vi "Get Hand Info p2.vi"(10 "Bid":u64, 11 "Hand":string) -> (3 "Hand Info":T1)   [LabVIEW 2023, in "d7.lvlib"]
uses:
  d7.lvlib
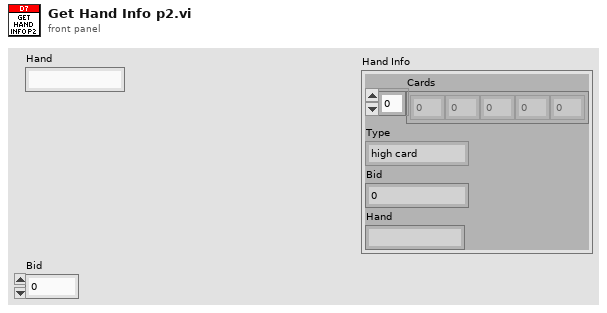
[diagram p1: front panel]
types:
  T1 = cluster{"Cards":i32[], "Type":enum16{"high card", "pair", "two pair", "3 of a kind", "full house", "4 of a kind", "5 of a kind"}, "Bid":u64, "Hand":string}
  T2 = enum16{"high card", "pair", "two pair", "3 of a kind", "full house", "4 of a kind", "5 of a kind"}
  T3 = cluster{i32[], enum16{"high card", "pair", "two pair", "3 of a kind", "full house", "4 of a kind", "5 of a kind"}, "Bid":u64, "Hand":string}
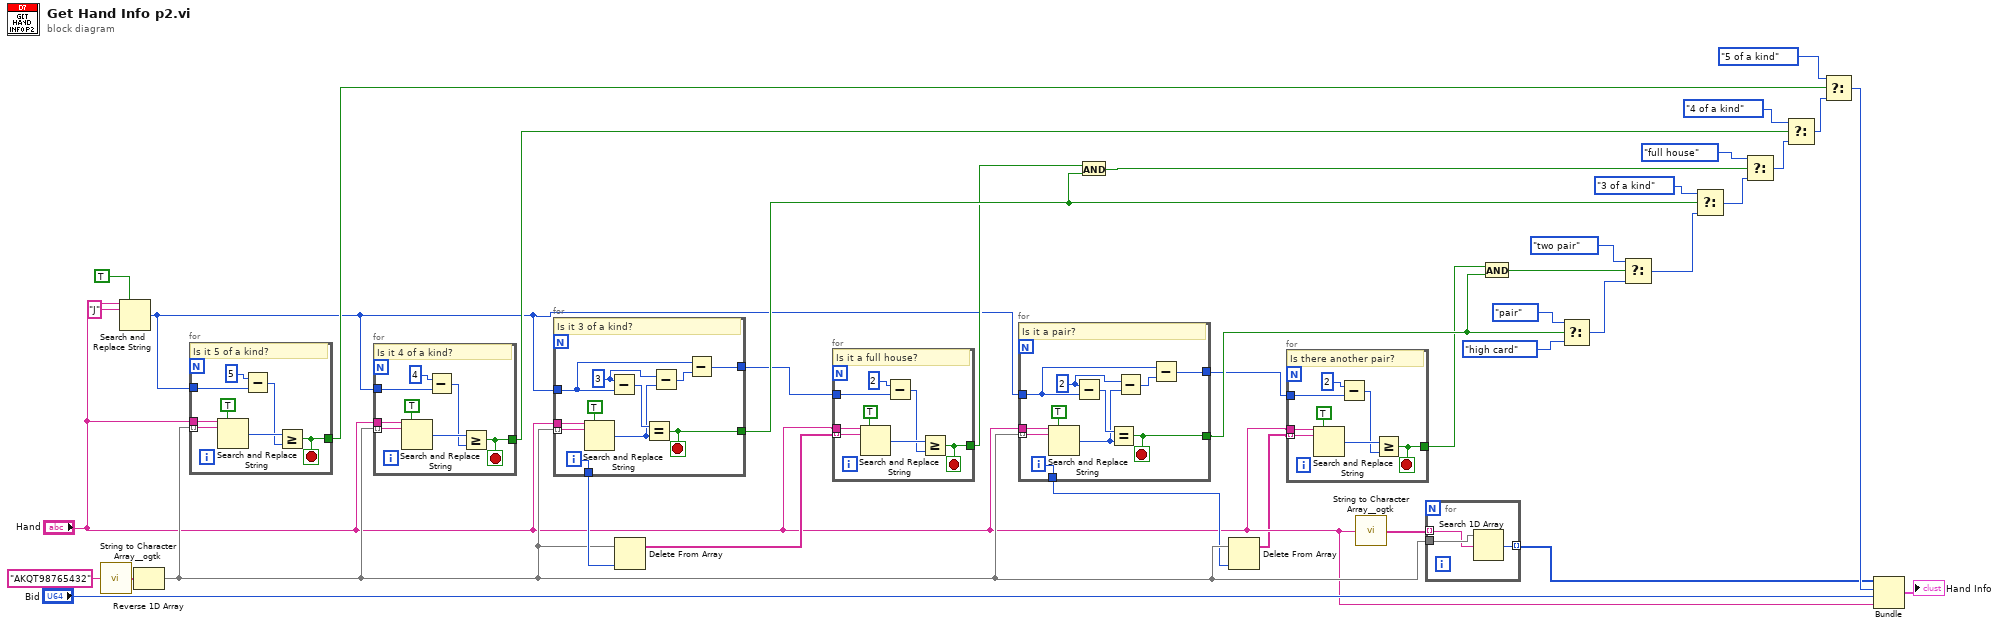
[diagram p0: block diagram]
diagram:
  n1 = call <userlib>:"String to Character Array__ogtk.vi"("Input String"="AKQT98765432" ("regular expression")) -> ("Character Array"=w27:string[])
  n2 = Search and Replace String(replace all?=TRUE ("replace all? (F)"), input string="Hand", search string="J" ("replace string (\"\")")) -> (number of replacements=w8:i32)  [unwired: 5 in, 3 out]
  n3 = Reverse 1D Array(array=w27) -> (reversed array=w9:string[])
  n4 = for {
    tunnel: w9 -> [w45] mode=indexing
    tunnel: "Hand" -> [w46]
    tunnel: [w43] -> w38
    tunnel: w8 -> [w42]
    stop <- w43 stop-if-true
    # "Is it 5 of a kind?"
    n5 = Search and Replace String(replace all?=TRUE ("replace all? (F)"), input string=w46, search string=w45) -> (number of replacements=w40:i32)  [unwired: 5 in, 3 out]
    n6 = Subtract(x=5 ("y"), y=w42) -> (x-y=w39:i32)
    n7 = Greater Or Equal?(x=w40, y=w39) -> (x >= y?=w43:bool)
  }
  n8 = for {
    tunnel: w9 -> [w53] mode=indexing
    tunnel: "Hand" -> [w54]
    tunnel: [w51] -> w15
    tunnel: w8 -> [w50]
    stop <- w51 stop-if-true
    # "Is it 4 of a kind?"
    n9 = Search and Replace String(replace all?=TRUE ("replace all? (F)"), input string=w54, search string=w53) -> (number of replacements=w48:i32)  [unwired: 5 in, 3 out]
    n10 = Subtract(x=4 ("y"), y=w50) -> (x-y=w47:i32)
    n11 = Greater Or Equal?(x=w48, y=w47) -> (x >= y?=w51:bool)
  }
  n12 = for {
    tunnel: w9 -> [w64] mode=indexing
    tunnel: "Hand" -> [w65]
    tunnel: [w62] -> w14
    tunnel: w8 -> [w56]
    tunnel: [w60] -> w13
    tunnel: [w55] -> w12
    i -> [w60]
    stop <- w62 stop-if-true
    w59 = 3 ("y")
    # "Is it 3 of a kind?"
    n13 = Search and Replace String(replace all?=TRUE ("replace all? (F)"), input string=w65, search string=w64) -> (number of replacements=w58:i32)  [unwired: 5 in, 3 out]
    n14 = Subtract(x=w59, y=w56) -> (x-y=w61:i32)
    n15 = Equal?(x=w61, y=w58) -> (x = y?=w62:bool)
    n16 = Subtract(x=w59, y=w58) -> (x-y=w57:i32)
    n17 = Subtract(x=w56, y=w57) -> (x-y=w55:i32)
  }
  n18 = Delete From Array(array=w9, index=w13) -> (array with subset deleted=w11:string[])  [unwired: 1 in, 1 out]
  n19 = for {
    tunnel: w11 -> [w72] mode=indexing
    tunnel: "Hand" -> [w73]
    tunnel: [w70] -> w10
    tunnel: w12 -> [w69]
    stop <- w70 stop-if-true
    # "Is it a full house?"
    n20 = Search and Replace String(replace all?=TRUE ("replace all? (F)"), input string=w73, search string=w72) -> (number of replacements=w67:i32)  [unwired: 5 in, 3 out]
    n21 = Subtract(x=2 ("y"), y=w69) -> (x-y=w66:i32)
    n22 = Greater Or Equal?(x=w67, y=w66) -> (x >= y?=w70:bool)
  }
  n23 = for {
    tunnel: w9 -> [w83] mode=indexing
    tunnel: "Hand" -> [w84]
    tunnel: [w81] -> w6
    tunnel: w8 -> [w75]
    tunnel: [w79] -> w7
    tunnel: [w74] -> w5
    i -> [w79]
    stop <- w81 stop-if-true
    w78 = 2 ("y")
    # "Is it a pair?"
    n24 = Search and Replace String(replace all?=TRUE ("replace all? (F)"), input string=w84, search string=w83) -> (number of replacements=w77:i32)  [unwired: 5 in, 3 out]
    n25 = Subtract(x=w78, y=w75) -> (x-y=w80:i32)
    n26 = Equal?(x=w80, y=w77) -> (x = y?=w81:bool)
    n27 = Subtract(x=w78, y=w77) -> (x-y=w76:i32)
    n28 = Subtract(x=w75, y=w76) -> (x-y=w74:i32)
  }
  n29 = And(x=w10, y=w14) -> (x .and. y?=w31:bool)
  n30 = Delete From Array(array=w9, index=w7) -> (array with subset deleted=w2:string[])  [unwired: 1 in, 1 out]
  n31 = for {
    tunnel: w2 -> [w91] mode=indexing
    tunnel: "Hand" -> [w92]
    tunnel: [w89] -> w4
    tunnel: w5 -> [w88]
    stop <- w89 stop-if-true
    # "Is there another pair?"
    n32 = Search and Replace String(replace all?=TRUE ("replace all? (F)"), input string=w92, search string=w91) -> (number of replacements=w86:i32)  [unwired: 5 in, 3 out]
    n33 = Subtract(x=2 ("y"), y=w88) -> (x-y=w85:i32)
    n34 = Greater Or Equal?(x=w86, y=w85) -> (x >= y?=w89:bool)
  }
  n35 = call <userlib>:"String to Character Array__ogtk.vi"("Input String"="Hand") -> ("Character Array"=w30:string[])
  n36 = for {
    tunnel: w30 -> [w94] mode=indexing
    tunnel: w9 -> [w95]
    tunnel: [w93] -> w29 mode=indexing
    n37 = Search 1D Array(1D array=w95, element=w94) -> (index of element=w93:i32)  [unwired: 1 in]
  }
  n38 = And(x=w4, y=w6) -> (x .and. y?=w24:bool)
  n39 = Select(t=T2."pair", s=w6, f=T2."high card") -> (s? t:f=w25:T2)
  n40 = Select(t=T2."two pair", s=w24, f=w25) -> (s? t:f=w26:T2)
  n41 = Select(t=T2."3 of a kind", s=w14, f=w26) -> (s? t:f=w35:T2)
  n42 = Select(t=T2."full house", s=w31, f=w35) -> (s? t:f=w36:T2)
  n43 = Select(t=T2."4 of a kind", s=w15, f=w36) -> (s? t:f=w37:T2)
  n44 = Select(t=T2."5 of a kind", s=w38, f=w37) -> (s? t:f=w34:T2)
  n45 = Bundle(w29, w34, "Bid"="Bid", "Hand"="Hand") -> (→"Hand Info":T3)  [unwired: 1 in]
